vi "Oxford Interface.vi"(8 "error in (no error)":errorcluster, 10 "Command":string, 11 "Address":refnum<visa-resource-name>) -> (0 "error out":errorcluster, 2 "Reply":string="ITC503 Version 1.11 (c) OXFORD 1997\r", 3 "Numeric reply":dbl format="%.2f")   [LabVIEW 2015]
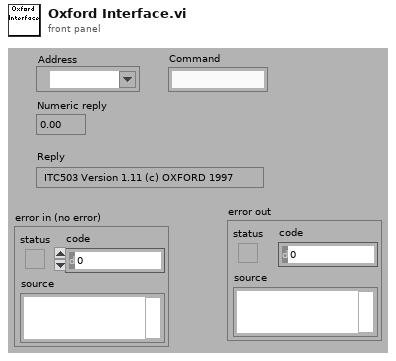
[diagram p1: front panel]
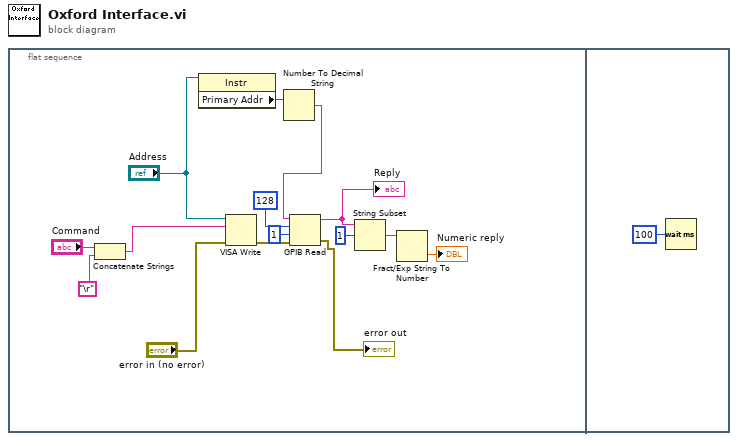
[diagram p0: block diagram]
diagram:
  n1 = flat-sequence {
    frame #0 {
      n2 = Concatenate Strings("Command", "\r") -> (w14:string)
      n3 = property class="Instr"(reference="Address") -> ("Primary Addr"=w7:u16)  [unwired: 1 in, 2 out]
      n4 = VISA Write(VISA resource name="Address", write buffer=w14, error in (no error)="error in (no error)") -> (error out=w6:errorcluster)  [unwired: 2 out]
      n5 = Number To Decimal String(number=w7) -> (decimal integer string=w4:string)  [unwired: 1 in]
      n6 = GPIB Read(0:w4, 1:u32 128 ("byte count"), 2:i16 1 ("mode (0)"), 3:w6) -> (5:w1:string, 7:→"error out":errorcluster)  [unwired: 1 in, 1 out]
      "Reply" <- w1
      n7 = String Subset(string=w1, offset (0)=1) -> (substring=w11:string)  [unwired: 1 out]
      n8 = Fract/Exp String To Number(string=w11) -> (number=→"Numeric reply":dbl)  [unwired: 4 out]
    }
    frame #1 {
      n9 = Wait (ms)(milliseconds to wait=u32 100) -> ()  [unwired: 1 out]
    }
  }
